vi "Tree Add Node.vi"(8 "error in (no error)":errorcluster, 9 "Usage":T1, 10 "Name":string, 11 "Tree DVR in":refnum<data-value>) -> (0 "error out":errorcluster, 2 "Node out":refnum<data-value>, 3 "Tree DVR out":refnum<data-value>)   [LabVIEW 2015, in "MDSplus.lvlib"]
doc: "Add a new node to the tree open for edit."
uses:
  <vilib>/MDSplus/Library/MDSplus.lvlib
  <vilib>/MDSplus/Classes/Tree_Class/Tree.lvclass
  <vilib>/MDSplus/Classes/Data_Class/TreeNode_Class/TreeNode.lvclass
  <vilib>/MDSplus/Library/Data/TreeNode/TreeNode Types.ctl
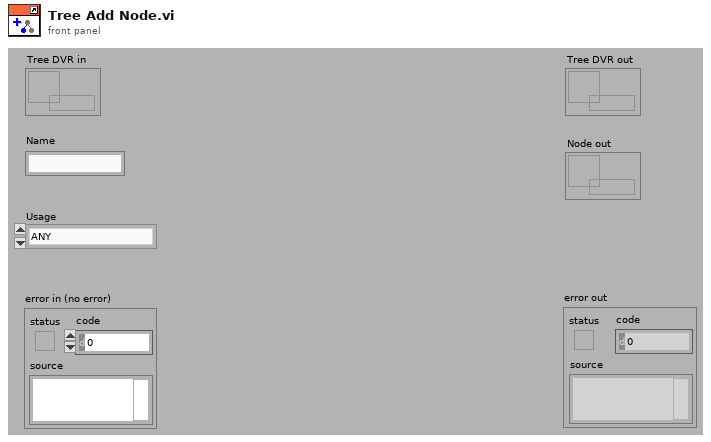
[diagram p1: front panel]
types:
  T1 = typedef "MDSplus.lvlib/TreeNode Types.ctl" = enum16{"ANY", "NONE", "STRUCTURE", "ACTION", "DEVICE", "DISPATCH", "NUMERIC", "SIGNAL", "TASK", "TEXT", "WINDOW", "AXIS", "SUBTREE", "COMPOUND_DATA"}
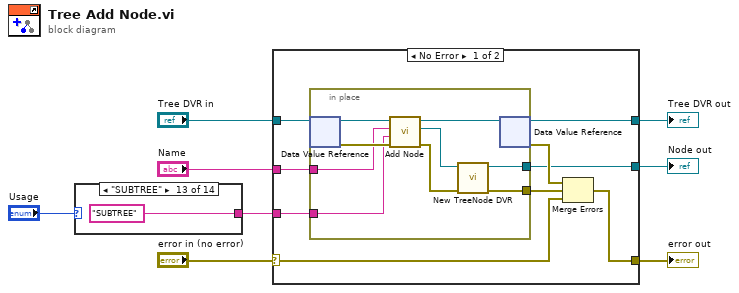
[diagram p0: block diagram]
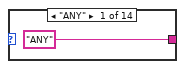
[diagram p2: hidden frame]
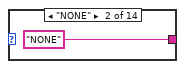
[diagram p3: hidden frame]
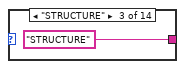
[diagram p4: hidden frame]
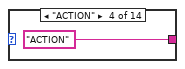
[diagram p5: hidden frame]
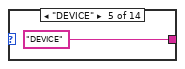
[diagram p6: hidden frame]
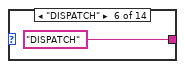
[diagram p7: hidden frame]
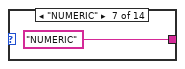
[diagram p8: hidden frame]
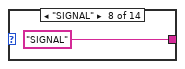
[diagram p9: hidden frame]
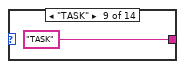
[diagram p10: hidden frame]
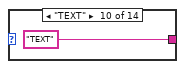
[diagram p11: hidden frame]
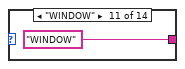
[diagram p12: hidden frame]
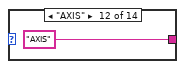
[diagram p13: hidden frame]
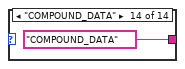
[diagram p14: hidden frame]
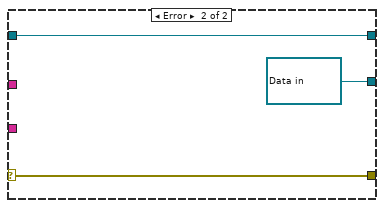
[diagram p15: hidden frame]
diagram:
  n1 = case shown="\"SUBTREE\"" "Usage" {
    tunnel: ["ANY" "NONE" "STRUCTURE" "ACTION" "DEVICE" "DISPATCH" "NUMERIC" "SIGNAL" "TASK" "TEXT" "WINDOW" "AXIS" "SUBTREE" "COMPOUND_DATA"] -> w1
    frame "ANY" {
    }
    frame "NONE" {
    }
    frame "STRUCTURE" {
    }
    frame "ACTION" {
    }
    frame "DEVICE" {
    }
    frame "DISPATCH" {
    }
    frame "NUMERIC" {
    }
    frame "SIGNAL" {
    }
    frame "TASK" {
    }
    frame "TEXT" {
    }
    frame "WINDOW" {
    }
    frame "AXIS" {
    }
    frame "SUBTREE" {
    }
    frame "COMPOUND_DATA" {
    }
  }
  n2 = case shown="No Error" "error in (no error)" {
    selector: "error in (no error)" -> [w30 w43]
    tunnel: "Tree DVR in" -> [w31 w42]
    tunnel: [w28 w43] -> w8
    tunnel: [w27 w42] -> w5
    tunnel: [w23 refnum<data-value> refnum ("TreeNode DVR out")] -> w3
    tunnel: "Name" -> [w26 _]
    tunnel: w1 -> [w25 _]
    frame No Error {
      n3 = in-place {
        in-place-border: [w32] -> w24
        in-place-border: [w34] -> w23
        in-place-border: w26 -> [w37]
        in-place-border: w25 -> [w36]
        n4 = in-place-dvr #1(w31) -> (w40:refnum<class "Tree.lvclass">, w38:errorcluster)
        n5 = call-dynamic "Add Node.vi"("error in (no error)"=w38, "Usage"=w36, "Name"=w37, "Tree in"=w40) -> ("error out"=w33:errorcluster, "Node out"=w35:refnum<class "TreeNode.lvclass">, "Tree out"=w39:refnum<class "Tree.lvclass">)  [unwired: 5 in]
        n6 = call <vilib>:"New TreeNode DVR.vi"("error in (no error)"=w33, "TreeNode in"=w35) -> ("error out"=w32:errorcluster, "TreeNode DVR out"=w34:refnum<data-value>)  [unwired: 8 in]
        n7 = in-place-dvr #1(w39) -> (w27:refnum<data-value>, w29:errorcluster)
      }
      n8 = Merge Errors(w29, w24, w30) -> (w28:errorcluster)
    }
    frame Error {
    }
  }
  "error out" <- w8
  "Tree DVR out" <- w5
  "Node out" <- w3
